vi "testlockin.vi"() -> ()   [LabVIEW 2016]
panel:
  in  "step":dbl
  in  "end":dbl
  in  "start":dbl
  in  "Channels: AO":T1={"AO amp (V)"=[1.0, 0.0, 0.0, 0.0, 0.0, 0.0, 0.0, 0.0], "AO DC (V)"=[0.0, 0.0, 0.0, 0.0, 0.0, 0.0, 0.0, 0.0], "AO f (Hz)"=[1.0, 1.0, 1.0, 1.0, 1.0, 1.0, 1.0, 1.0], "AO phi (deg)"=[0.0, 0.0, 0.0, 0.0, 0.0, 0.0, 0.0, 0.0], "function"=[enum."Triangle Wave", enum."Sine Wave", enum."Sine Wave", enum."Sine Wave", enum."Sine Wave", enum."Sine Wave", enum."Sine Wave", enum."Sine Wave"]} {"AO DC (V)" format="%#_6p"; "AO amp (V)" format="%#_6p"}
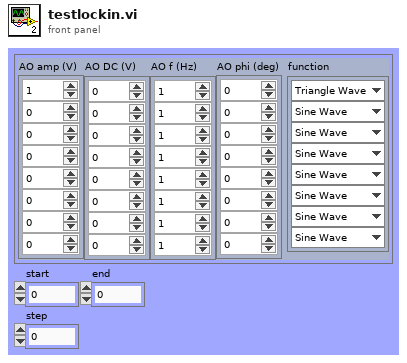
[diagram p1: front panel]
types:
  T1 = cluster{"AO amp (V)":dbl[], "AO DC (V)":dbl[], "AO f (Hz)":dbl[], "AO phi (deg)":dbl[], "function":enum16{"Sine Wave", "Triangle Wave", "Square Wave", "Sawtooth Wave"}[]}
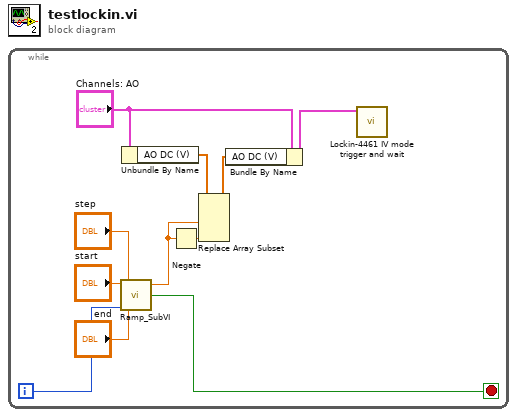
[diagram p0: block diagram]
diagram:
  n1 = while {
    i -> [w11]
    stop <- w10 stop-if-true
    n2 = call <userlib>:"Ramp_SubVI.vi"("index"=w11, "step"="step", "end"="end", "start"="start") -> ("Stop?"=w10:bool, "Numeric"=w5:dbl)  [unwired: 1 in]
    n3 = Unbundle By Name("Channels: AO") -> ("AO DC (V)"=w7:dbl[])
    n4 = Negate(x=w5) -> (-x=w1:dbl)
    n5 = Replace Array Subset(array=w7, new element #1=w5, new element #2=w1) -> (w6:dbl[])  [unwired: 2 in]
    n6 = Bundle By Name(cluster="Channels: AO", "AO DC (V)"=w6) -> (w9:T1)
    n7 = call "Lockin-4461 IV mode trigger and wait.vi"("Channels: AO"=w9) -> ()  [unwired: 10 in, 1 out]
  }
